vi "Position_PID.vi"(1 "Target_Position":dbl, 2 "Encoder":dbl) -> (0 "PWM":dbl)   [LabVIEW 2018]
uses:
  Global_variables.vi
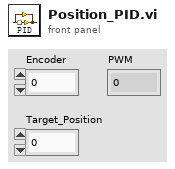
[diagram p1: front panel]
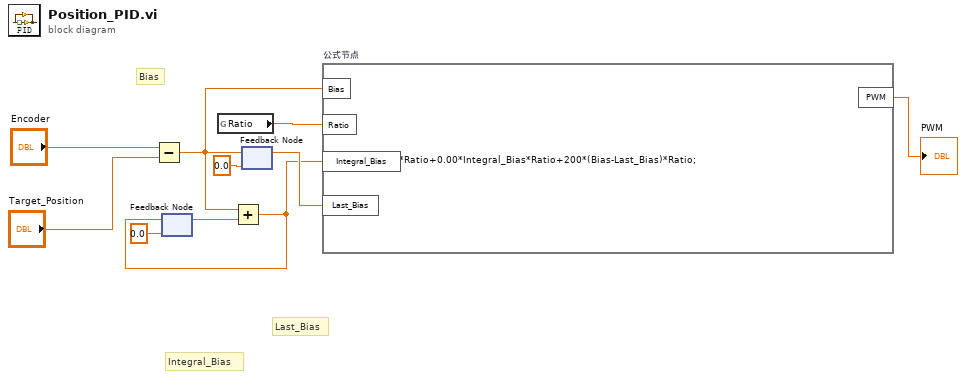
[diagram p0: block diagram]
diagram:
  # "Last_Bias"
  # "Integral_Bias"
  # "Bias"
  n1 = Subtract(x="Encoder", y="Target_Position") -> (x-y=w3:dbl)
  n2 = feedback #1(0.0) -> (w7:dbl)
  n3 = global read "Global_variables.vi" "Ratio"() -> (w2:dbl)
  n4 = Add(x=w3, y=w7) -> (x+y=w4:dbl)
  n5 = feedback-in #1(w4) -> ()
  n6 = feedback-in #2(w3) -> ()
  n7 = feedback #2(0.0) -> (w5:dbl)
  n8 = formula code="PWM=90*Bias*Ratio+0.00*Integral_Bias*Ratio+200*(Bias-Last_Bias)*Ratio;" "公式节点"("Bias"=w3, "Ratio"=w2, "Integral_Bias"=w4, "Last_Bias"=w5) -> ("PWM"=→"PWM":dbl)
